vi "Fit Transform.vi"(7 "Type X":T1(ring), 8 "error in (no error)":errorcluster caption="entrée d'erreur (pas d'erreur)", 9 "y":string[][](array[string]), 10 "X":string[][](array[string]), 11 "SkewedChi2Sampler.lvclass":refnum<class "SkewedChi2Sampler.lvclass">) -> (0 "error in (no error)":errorcluster caption="entrée d'erreur (pas d'erreur)", 2 "Data":T2, 3 "SkewedChi2Sampler.lvclass":refnum<class "SkewedChi2Sampler.lvclass">)   [LabVIEW 2020, in "SkewedChi2Sampler.lvclass"]
doc: "Fit to data, then transform it.\n\nFits transformer to X and y with optional parameters fit_params and returns a transformed version of X.\n\nReturns : \n\n- X_new : ndarray array of shape (n_samples, n_features_new)\nTransformed array."
uses:
  SkewedChi2Sampler.lvclass
  SkewedChi2Sampler.lvclass/SkewedChi2Sampler.ctl
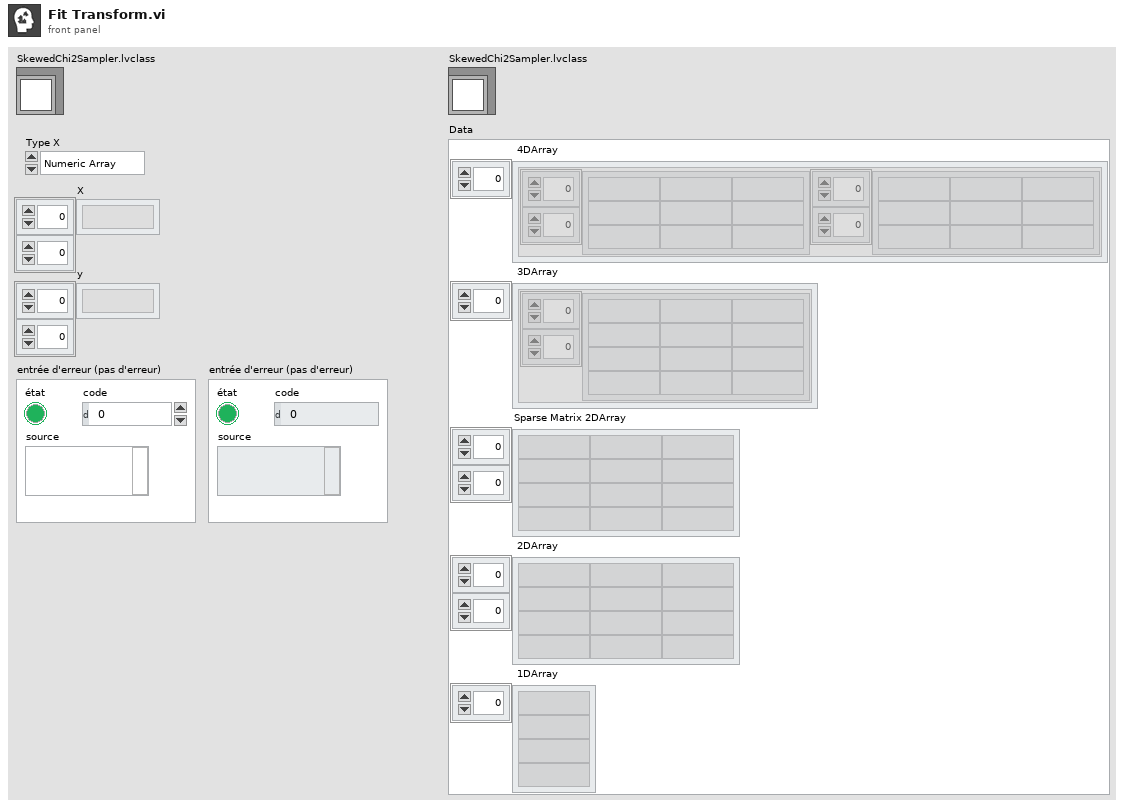
[diagram p1: front panel]
types:
  T1 = enum16{"Numeric Array", "String Array", "Sparse"}
  T2 = cluster{" 4DArray":cluster{"1":string[][], "2":string[][]}[], " 3DArray":cluster{"Tableau":string[][]}[], "Sparse Matrix 2DArray":string[][], " 2DArray":string[][], " 1DArray":string[]}
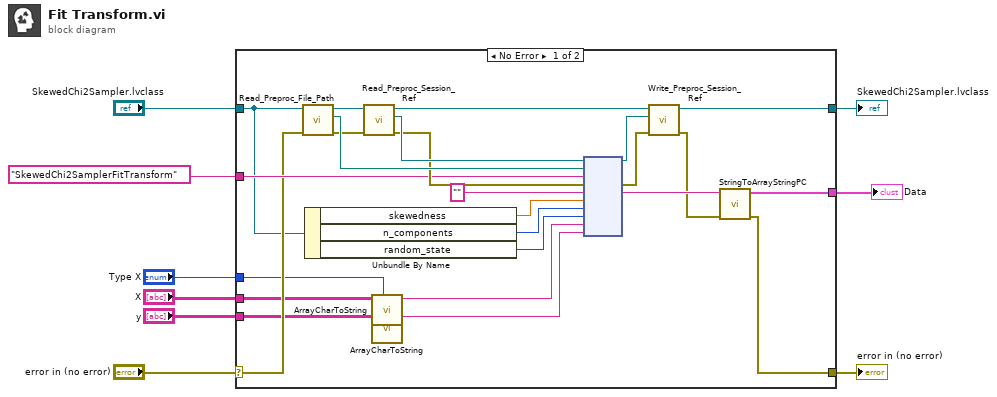
[diagram p0: block diagram]
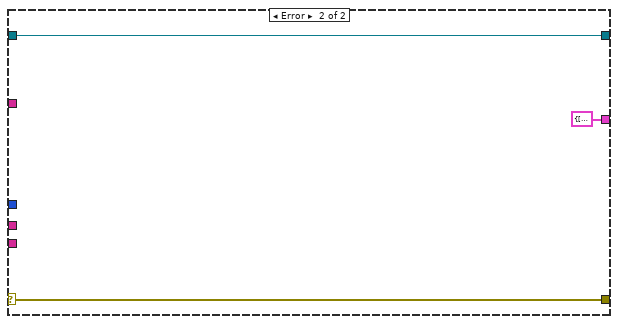
[diagram p2: hidden frame]
diagram:
  n1 = case shown="No Error" "error in (no error)" {
    selector: "error in (no error)" -> [w22 w37]
    tunnel: [w16 w37] -> w8
    tunnel: [w19 w36] -> w6
    tunnel: "SkewedChi2Sampler.lvclass" -> [w21 w36]
    tunnel: "SkewedChi2SamplerFitTransform" ("Fonction") -> [w23 _]
    tunnel: "X" -> [w14 _]
    tunnel: "y" -> [w12 _]
    tunnel: [w15 T2 {" 4DArray"=[], " 3DArray"=[], "Sparse Matrix 2DArray"=[], " 2DArray"=[], " 1DArray"=[]} ("Data")] -> w2
    tunnel: "Type X" -> [w10 _]
    frame No Error {
      n2 = call-dynamic "Read_Preproc_File_Path.vi"("error in (no error)"=w22, "Python in"=w21) -> ("error out"=w29:errorcluster, "File_Path"=w32:path, "Python out"=w34:refnum<class "SkewedChi2Sampler.lvclass">)  [unwired: 7 in]
      n3 = Unbundle By Name(w21) -> ("skewedness"=w25:dbl, "n_components"=w24:i32, "random_state"=w20:i32)
      n4 = call-dynamic "Read_Preproc_Session_Ref.vi"("error in (no error)"=w29, "Python in"=w34) -> ("error out"=w30:errorcluster, "Session_ref"=w31:refnum<k35>, "Python out"=w33:refnum<class "SkewedChi2Sampler.lvclass">)  [unwired: 7 in]
      n5 = call "ArrayCharToString.vi"("Type"=w10, "TAB"=w14) -> ("Instruction"=w13:string)  [unwired: 9 in]
      n6 = call "ArrayCharToString.vi"("TAB"=w12) -> ("Instruction"=w11:string)  [unwired: 10 in]
      n7 = node(w31, w32, w23, w30, "", w25, w24, w20, w13, w11) -> (w26:refnum<k35>, w28:errorcluster, w18:string)  [unwired: 5 in, 2 out]
      n8 = call-dynamic "Write_Preproc_Session_Ref.vi"("error in (no error)"=w28, "Session_ref"=w26, "Python in"=w33) -> ("error out"=w17:errorcluster, "Python out"=w19:refnum<class "SkewedChi2Sampler.lvclass">)  [unwired: 7 in]
      n9 = call "StringToArrayStringPC.vi"("sortie d'erreur"=w17, "Return value"=w18) -> ("sortie d'erreur"=w16:errorcluster, "Data"=w15:T2)  [unwired: 8 in]
    }
    frame Error {
    }
  }
  "error in (no error)" <- w8
  "SkewedChi2Sampler.lvclass" <- w6
  "Data" <- w2
